vi "ViewTDMSData.vi"(8 "Error In":errorcluster, 11 "file path":path) -> (0 "Error Out":errorcluster)   [LabVIEW 2018]
doc: "This VI sends a message to load the plugin into the module."
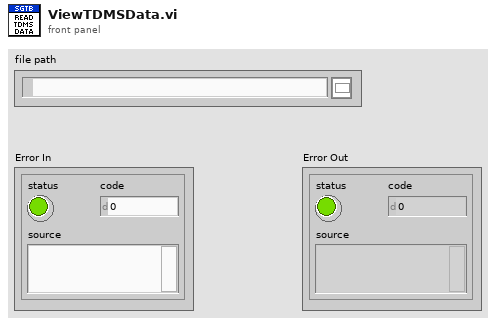
[diagram p1: front panel]
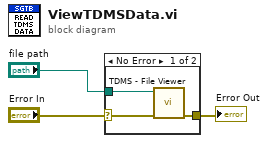
[diagram p0: block diagram]
diagram:
  n1 = case shown="No Error" "Error In" {
    selector: "Error In" -> [w5 w7]
    tunnel: [w6 w7] -> w3
    tunnel: "file path" -> [w4 _]
    frame No Error {
      n2 = call <vilib>:"TDMS - File Viewer.vi"("error in (no error)"=w5, "file path"=w4) -> ("error out"=w6:errorcluster)  [unwired: 4 in, 1 out]
    }
    frame Error {
    }
  }
  "Error Out" <- w3
